vi "Write Power Meter Reverse.vi"(10 "Power Meter.lvclass":refnum<class "Power Meter.lvclass">, 11 "AM-AM in":refnum<class "AM-AM.lvclass">) -> (3 "AM-AM out":refnum<class "AM-AM.lvclass">)   [LabVIEW 2020, in "AM-AM.lvclass"]
uses:
  AM-AM.lvclass
  Instruments/Power Meter/Power Meter.lvclass
  AM-AM.lvclass/AM-AM.ctl
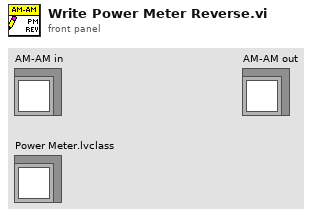
[diagram p1: front panel]
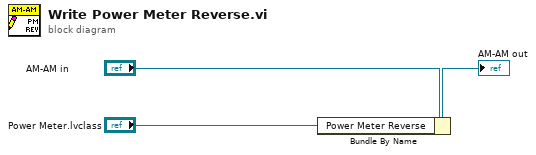
[diagram p0: block diagram]
diagram:
  n1 = Bundle By Name(cluster="AM-AM in", "Power Meter Reverse"="Power Meter.lvclass") -> (→"AM-AM out":refnum<class "AM-AM.lvclass">)
